vi "Start_Experiment.vi"   [LabVIEW 2016]
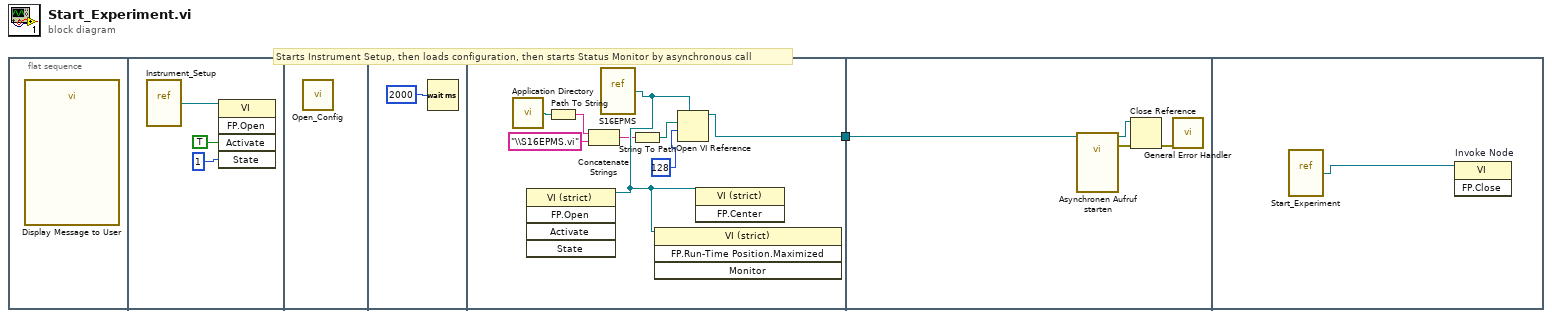
[diagram p0: block diagram]
diagram:
  # "Starts Instrument Setup, then loads configuration, then starts Status Monitor by asynchronous call"
  n1 = flat-sequence {
    tunnel: [w6] -> w1
    tunnel: w1 -> [w14]
    frame #0 {
      n2 = call "Display Message to User"() -> ()  [unwired: 10 in, 2 out]
    }
    frame #1 {
      n3 = vi-ref "Instrument_Setup.vi"() -> (w4:refnum<vi>)
      n4 = invoke class="VI" method="FP.Open"(reference=w4, "Activate"=TRUE, "State"=1) -> ()  [unwired: 2 in, 5 out]
    }
    frame #2 {
      n5 = call "Open_Config.vi"() -> ()  [unwired: 12 in]
    }
    frame #3 {
      n6 = Wait (ms)(milliseconds to wait=2000) -> ()  [unwired: 1 out]
    }
    frame #4 {
      n7 = call <vilib>:"Application Directory.vi"() -> ("Application Directory"=w7:path)
      n8 = Path To String(path=w7) -> (string=w8:string)
      n9 = Concatenate Strings(w8, "\\S16EPMS.vi") -> (w9:string)
      n10 = vi-ref "S16EPMS.vi"() -> (w13:refnum<vi>)
      n11 = invoke class="VI (strict)" method="FP.Open"(reference=w13) -> ()  [unwired: 4 in, 5 out]
      n12 = String To Path(string=w9) -> (path=w11:path)
      n13 = invoke class="VI (strict)" method="FP.Run-Time Position.Maximized"(reference=w13) -> ()  [unwired: 3 in, 4 out]
      n14 = Open VI Reference ("VI-Referenz öffnen")(type specifier VI Refnum (for type only)=w13, vi path=w11, options=128) -> (vi reference=w6:refnum<vi>)  [unwired: 3 in, 1 out]
      n15 = invoke class="VI (strict)" method="FP.Center"(reference=w13) -> ()  [unwired: 2 in, 3 out]
    }
    frame #5 {
      n16 = call-by-ref "Asynchronen Aufruf starten"(reference=w14) -> (reference out=w17:refnum<vi>, error out=w16:errorcluster)  [unwired: 13 in]
      n17 = Close Reference(reference=w17, error in (no error)=w16) -> (error out=w15:errorcluster)
      n18 = call <vilib>:"General Error Handler.vi"("error in (no error)"=w15) -> ()  [unwired: 10 in, 5 out]
    }
    frame #6 {
      n19 = vi-ref "Start_Experiment.vi"() -> (w18:refnum<vi>)
      n20 = invoke on="Invoke Node" class="VI" method="FP.Close"(reference=w18) -> ()  [unwired: 2 in, 3 out]
    }
  }
